vi "test Empty Filters.vi"(8 "error in (no error)":errorcluster, 11 "BM Filters in":refnum<class "BM Filters.lvclass">) -> (0 "error out":errorcluster, 3 "BM Filters out":refnum<class "BM Filters.lvclass">)   [LabVIEW 2016, in "BM Filters.lvclass"]
uses:
  BM Filters.lvclass
  1553 Board/1553 Board.lvclass
  PPLs/FPGA Interface.lvlibp/FPGA Interface/FPGA Interface.lvclass
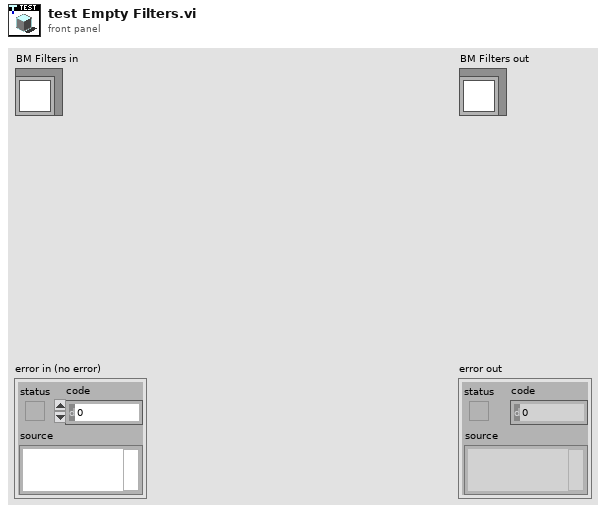
[diagram p1: front panel]
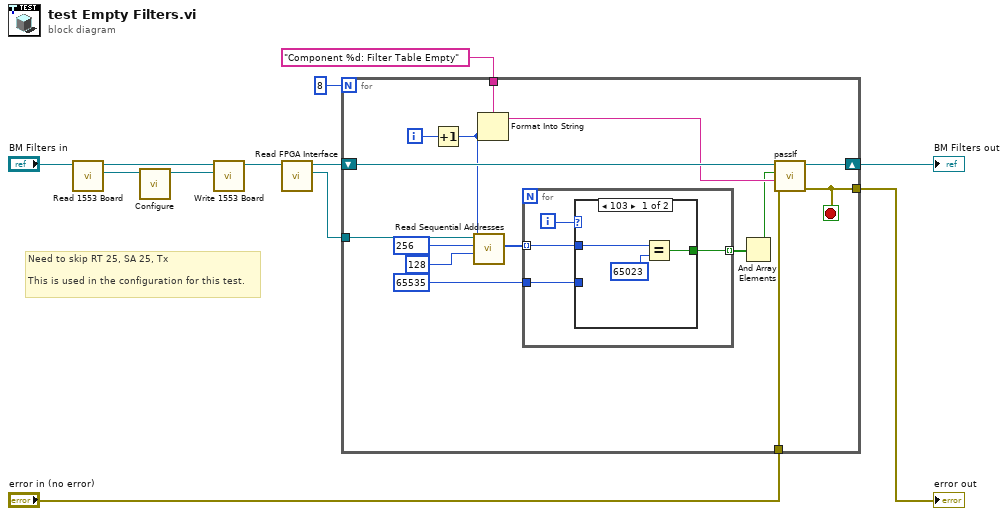
[diagram p0: block diagram]
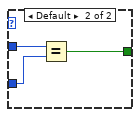
[diagram p2: hidden frame]
diagram:
  # "Need to skip RT 25, SA 25, Tx\n\nThis is used in the configuration for this test."
  n1 = call-dynamic "Read 1553 Board.vi"("1553 Test in"="BM Filters in") -> ("1553 Board"=w10:refnum<class "1553 Board.lvclass">, "1553 Test out"=w12:refnum<class "BM Filters.lvclass">)  [unwired: 8 in, 1 out]
  n2 = call-dynamic "Configure.vi"("1553 Board in"=w10) -> ("1553 Board out"=w9:refnum<class "1553 Board.lvclass">)  [unwired: 9 in, 1 out]
  n3 = call-dynamic "Write 1553 Board.vi"("1553 Board"=w9, "1553 Test in"=w12) -> ("1553 Test out"=w3:refnum<class "BM Filters.lvclass">)  [unwired: 8 in, 1 out]
  n4 = call-dynamic "Read FPGA Interface.vi"("1553 Test in"=w3) -> ("FPGA Interface"=w1:refnum<class "FPGA Interface.lvclass">, "1553 Test out"=w2:refnum<class "BM Filters.lvclass">)  [unwired: 8 in, 1 out]
  n5 = for {
    N: 8 -> [_]
    shift-right: [w24] -> w7
    shift-left: w2 -> [w25]
    tunnel: "Component %d: Filter Table Empty" ("custom report message (\"\")") -> [w26]
    tunnel: "error in (no error)" -> [w23]
    tunnel: [w22] -> w4
    tunnel: w1 -> [w20]
    i -> [w27]
    stop <- w22 stop-if-true
    n6 = Increment(x=w27) -> (x+1=w19:i32)
    n7 = call-dynamic "Read Sequential Addresses.vi"("Target IC (1-8)"=w19, "Addresses to Read"=u16 128, "Starting Address"=u16 256, "FPGA Interface in"=w20) -> ("Data"=w16:u16[])  [unwired: 6 in, 1 out]
    n8 = Format Into String(format string=w26, w19) -> (resulting string=w21:string)  [unwired: 2 in, 1 out]
    n9 = for {
      tunnel: w16 -> [w30] mode=indexing
      tunnel: u16 65535 -> [w29]
      tunnel: [w28] -> w14 mode=indexing
      i -> [w31]
      n10 = case shown="103" w31 {
        tunnel: w30 -> [w34 w37]
        tunnel: w29 -> [_ w36]
        tunnel: [w32 w35] -> w28
        frame 103 {
          n11 = Equal?(x=w34, y=u16 65023) -> (x = y?=w32:bool)
        }
        frame Default {
          n12 = Equal?(x=w37, y=w36) -> (x = y?=w35:bool)
        }
      }
    }
    n13 = And Array Elements(Boolean array=w14) -> (logical AND=w13:bool)
    n14 = call-dynamic "passIf.vi"("error in (no error)"=w23, "message (\"\")"=w21, "pass"=w13, "TestCase in"=w25) -> ("error out"=w22:errorcluster, "TestCase out"=w24:refnum<class "BM Filters.lvclass">)  [unwired: 6 in]
  }
  "error out" <- w4
  "BM Filters out" <- w7
